vi "test_user_event_no_queue.vi"() -> ()   [LabVIEW 2025]
panel:
  out "slide voltage":dbl format="%#_13g"
  in  "stop":bool
  in  "Slide1":dbl(slide) scale=0.0..10.0
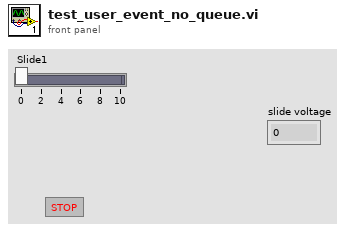
[diagram p1: front panel]
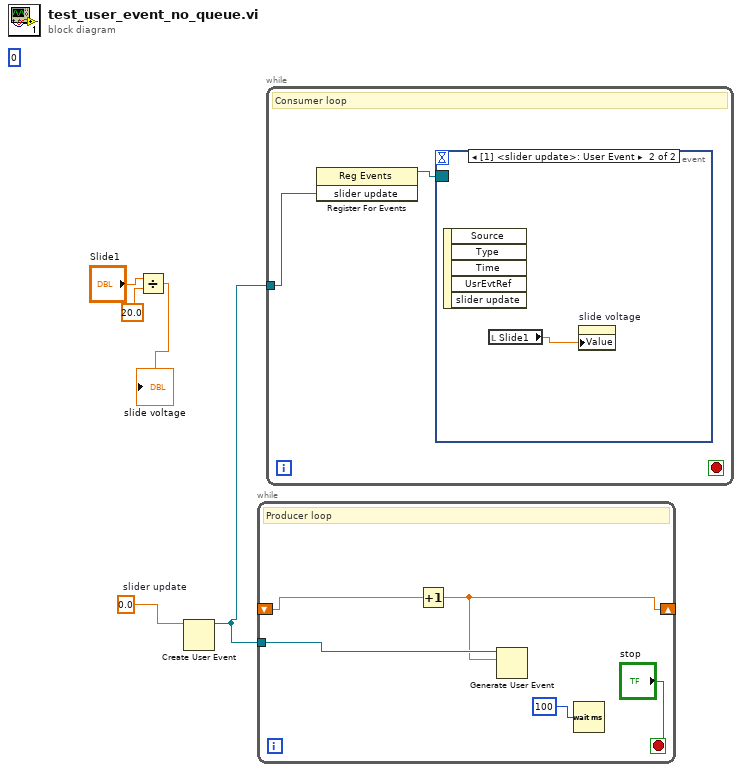
[diagram p0: block diagram]
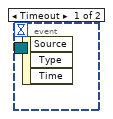
[diagram p2: hidden frame]
diagram:
  (unwired) 0
  w5 = 0.0  # slider update
  n1 = Divide(x="Slide1", y=20.0) -> (x/y=→"slide voltage":dbl)
  n2 = Create User Event(user event datatype=w5) -> (user event=w4:refnum<user-event>)  [unwired: 1 in, 1 out]
  n3 = while {
    shift-right: [w8] -> _
    shift-left: _ -> [w10]
    tunnel: w4 -> [w9]
    stop <- "stop" stop-if-true
    # "Producer loop"
    n4 = Increment(x=w10) -> (x+1=w8:dbl)
    n5 = Generate User Event(user event=w9, event data cluster=w8) -> ()  [unwired: 2 in, 2 out]
    n6 = Wait (ms)(milliseconds to wait=u32 100) -> ()  [unwired: 1 out]
  }
  n7 = while {
    tunnel: w4 -> [w12]
    stop <- _ stop-if-true
    # "Consumer loop"
    n8 = register-events(w12) -> (reference out=w11:refnum<event-registration>)  [unwired: 2 in, 1 out]
    n9 = event shown="[1] <slider update>: User Event" {
      selector: w11 -> [_ _]
      dyn-events: _ -> [_ _]
      timeout: _ -> [_ _]
      event Timeout {
        n10 = event-data() -> ()  [unwired: 1 in, 3 out]
      }
      event User Event {
        n11 = event-data() -> ()  [unwired: 1 in, 5 out]
        n12 = local read "Slide1"() -> (w13:dbl)
        n13 = property on="slide voltage" class="DigNum (strict)"("Value"=w13) -> ()  [unwired: 2 in, 2 out]
      }
    }
  }
